vi "Reset.vi"(8 "error in (no error)":errorcluster, 11 "VISA resource name":refnum<visa-resource-name>) -> (0 "error out":errorcluster, 3 "VISA resource name out":refnum<visa-resource-name>)   [LabVIEW 2015, in "Voltech PM1000+.lvlib"]
doc: "Resets the instrument and then sends a set of default setup commands to the instrument."
uses:
  <instrlib>/Voltech PM1000+/Voltech PM1000+.lvlib
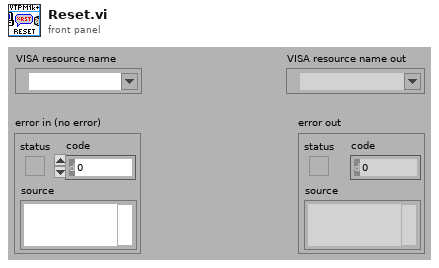
[diagram p1: front panel]
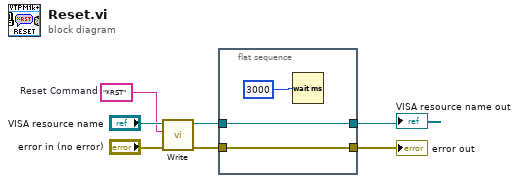
[diagram p0: block diagram]
diagram:
  w3 = "*RST"  # Reset Command
  n1 = call <instrlib>:"Write.vi"("error in (no error)"="error in (no error)", "Write Buffer"=w3, "VISA resource name"="VISA resource name") -> ("error out"=w4:errorcluster, "VISA resource name out"=w5:refnum<visa-resource-name>)  [unwired: 7 in]
  n2 = flat-sequence {
    tunnel: [w10] -> w2
    tunnel: w5 -> [w10]
    tunnel: [w9] -> w1
    tunnel: w4 -> [w9]
    frame #0 {
      n3 = Wait (ms)(milliseconds to wait=3000) -> ()  [unwired: 1 out]
    }
  }
  "error out" <- w1
  "VISA resource name out" <- w2
